vi "Universal_Virtual_Filter.vi"() -> ()   [LabVIEW 2018]
uses:
  Global_Signal.vi
  Global_Noise.vi
  <vilib>/measure/macond.llb/IIR Filter for 1 Chan.vi
  <vilib>/measure/macond.llb/FIR Filter for 1 Chan.vi
  <vilib>/measure/NI_MAPro.lvlib
panel:
  in  "Reset":bool
  in  "Power":bool
  out "Running":bool
  in  "Pause":bool=TRUE
  out "Signal_Graphics":waveform(dbl)(graph)
  in  "FIR_Advanced":T1={"Passband_Gain(dB)"=-3.0, "Stopband_Gain(dB)"=-60.0, "Ruler"=FALSE, "Windows"=0}
  in  "FIR_Basic":T2={"Design_Type"=0, "Passband"=0, "Taps"=50, "Lowest_Passband"=100.0, "Highest_Passband"=0.0, " Lowest_Stopband"=200.0, "Highest_Stopband"=0.0} {"Passband" items=["Lowpass", "Highpass", "Bandpass", "Bandstop"]; "Design_Type" items=["Off", "FIR by Specification", "Equi-ripple FIR", "Windowed FIR"]}
  in  "IIR_Advanced":T3={"Lowest_Passband"=100.0, "Highest_Passband"=0.0, "Lowest_Stopband"=200.0, "Highest_Stopband"=0.0, "Passband_Gain(dB)"=-3.0, "Stopband_Gain(dB)"=-60.0, "Ruler"=FALSE}
  in  "IIR_Basic":T4={"Design_Type"=0, "Passband"=0, "Rank"=2, "Low_Cutoff_Frequency"=100.0, "High_Cutoff_Frequency"=0.0, "Passband_Ripple"=1.0, " Stopband_Attenuation"=60.0} {"Passband" items=["Lowpass", "Highpass", "Bandpass", "Bandstop"]; "Design_Type" items=["Off", "Butterworth", "Chebyshev", "Inverse_Chebyshev", "Elliptic", "Bessel"]}
  out "Noised_Graphics":waveform(dbl)(graph)
  in  "Filter_Style":u16(ring) items=["IIR", "FIR"]
  out "Filtered_Graphics":waveform(dbl)(graph)
  # "Virtual Filter"
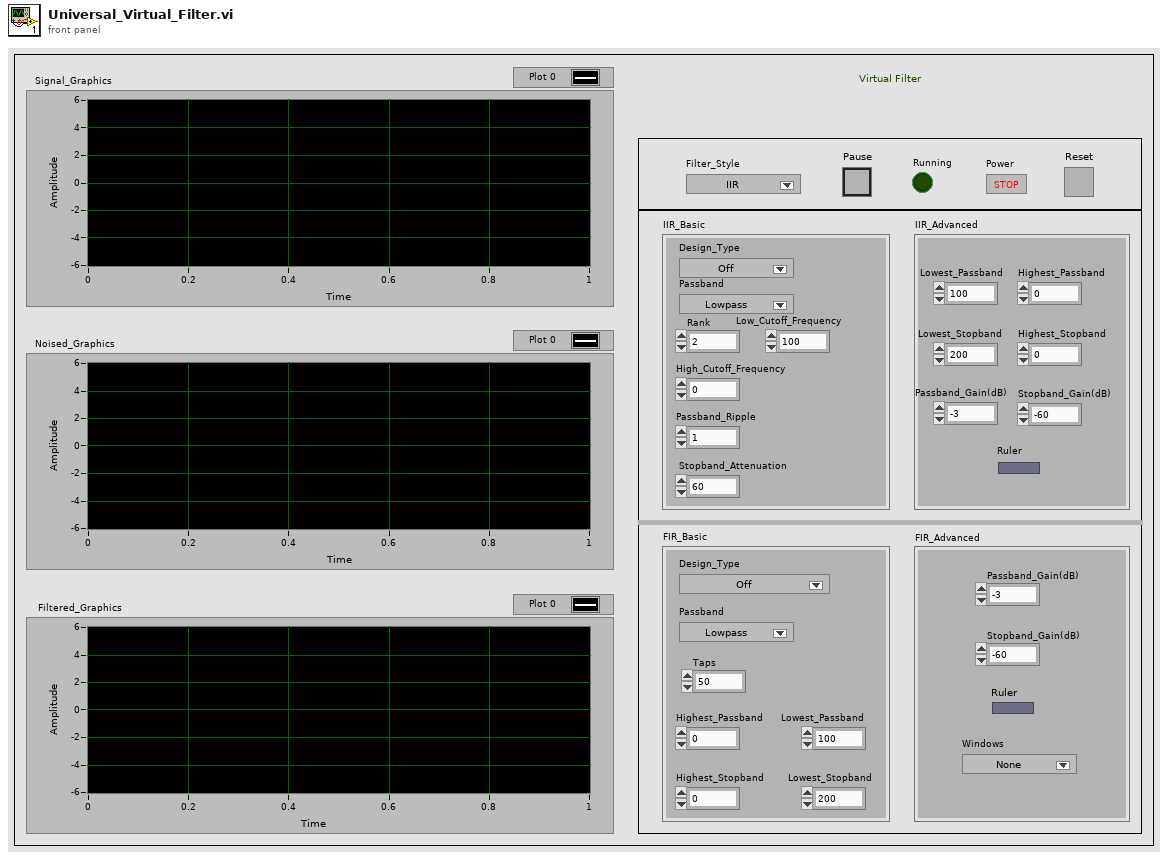
[diagram p1: front panel]
types:
  T1 = cluster{"Passband_Gain(dB)":dbl, "Stopband_Gain(dB)":dbl, "Ruler":bool, "Windows":u16}
  T2 = cluster{"Design_Type":u16, "Passband":u16, "Taps":i32, "Lowest_Passband":dbl, "Highest_Passband":dbl, " Lowest_Stopband":dbl, "Highest_Stopband":dbl}
  T3 = cluster{"Lowest_Passband":dbl, "Highest_Passband":dbl, "Lowest_Stopband":dbl, "Highest_Stopband":dbl, "Passband_Gain(dB)":dbl, "Stopband_Gain(dB)":dbl, "Ruler":bool}
  T4 = cluster{"Design_Type":u16, "Passband":u16, "Rank":i32, "Low_Cutoff_Frequency":dbl, "High_Cutoff_Frequency":dbl, "Passband_Ripple":dbl, " Stopband_Attenuation":dbl}
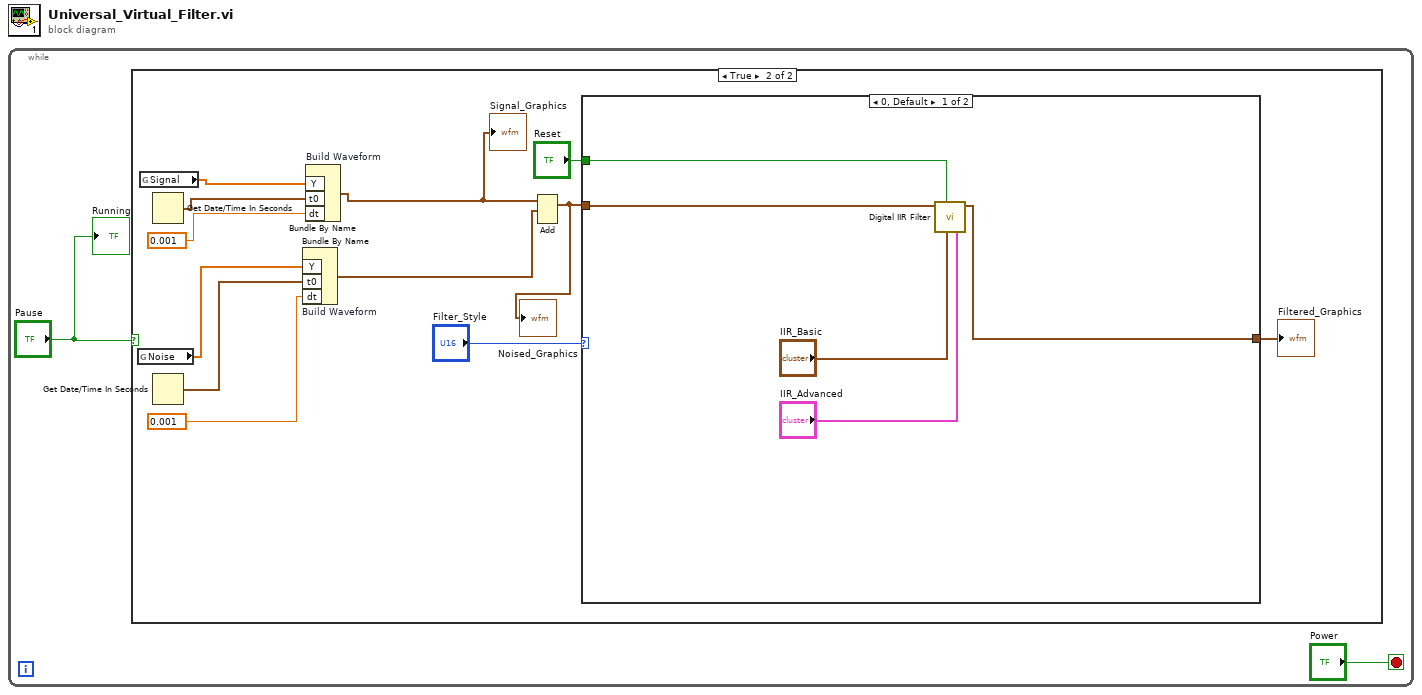
[diagram p0: block diagram]
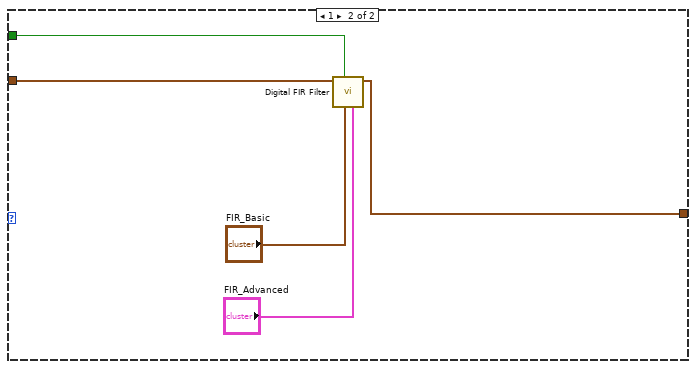
[diagram p3: hidden frame]
diagram:
  n1 = while {
    stop <- "Power" stop-if-true
    n2 = case shown="True" "Pause" {
      frame False {
      }
      frame True {
        n3 = global read "Global_Noise.vi" "Noise"() -> (w6:dbl[])
        n4 = global read "Global_Signal.vi" "Signal"() -> (w11:dbl[])
        n5 = Get Date/Time In Seconds() -> (seconds since 1Jan1904=w10:timestamp)
        n6 = Get Date/Time In Seconds() -> (seconds since 1Jan1904=w8:timestamp)
        n7 = Bundle By Name "Build Waveform"("Y"=w6, "t0"=w8, "dt"=0.001) -> (w5:waveform(dbl))  [unwired: 1 in]
        n8 = Bundle By Name "Build Waveform"("Y"=w11, "t0"=w10, "dt"=0.001) -> (w4:waveform(dbl))  [unwired: 1 in]
        "Signal_Graphics" <- w4
        n9 = Add(1:w5, 2:w4) -> (0:w3:waveform(dbl))  [unwired: 1 in, 1 out]
        "Noised_Graphics" <- w3
        n10 = case shown="0, Default" "Filter_Style" {
          tunnel: [w19 w24] -> w13
          tunnel: "Reset" -> [w16 w21]
          tunnel: w3 -> [w15 w20]
          frame 0, Default {
            n11 = call-poly <vilib>:"Digital IIR Filter.vi"("optional IIR filter specifications"="IIR_Advanced", "IIR filter specifications"="IIR_Basic", "reset filter"=w16, "signal in"=w15) -> ("signal out"=w19:waveform(dbl))  [unwired: 5 in, 2 out]
          }
          frame 1 {
            n12 = call-poly <vilib>:"Digital FIR Filter.vi"("optional FIR filter specifications"="FIR_Advanced", "FIR filter specifications"="FIR_Basic", "reset filter"=w21, "signal in"=w20) -> ("signal out"=w24:waveform(dbl))  [unwired: 5 in, 2 out]
          }
        }
        "Filtered_Graphics" <- w13
      }
    }
    "Running" <- "Pause"
  }
